vi "_Subscr.Ver Test Module2.vi"() -> ()   [LabVIEW 2024, in "EQMF.lvlib" / "Subscription.lvlib"]
uses:
  Subscription.lvlib
  Subscr.Subscription Request Info.ctl
  Queues/Q.Element.ctl
  Subscription.lvclass
  Queues/Queue Utils.lvlib
panel:
  out "SubScrReq":T1[](array[typedef])
  in  "stop":bool
  in  "Bool":bool
  in  "Str":string
  in  "Host Q":string="Module 1"
  out "Bool  Subsc":bool
  out "Str Subsc":string
  in  "Subscribe to Bool":bool
  in  "Subscribe to Str":bool
  in  "Local Q":string="Module 2"
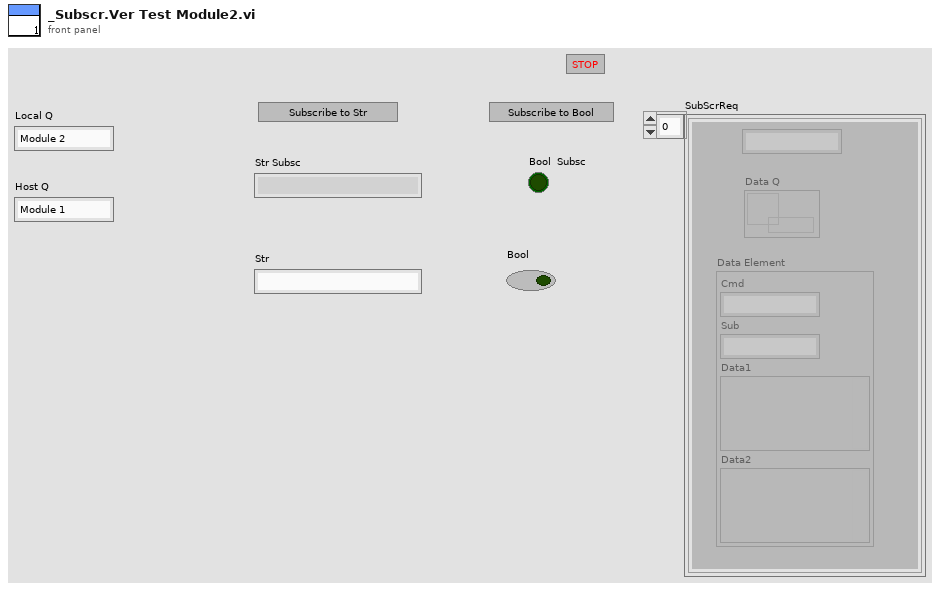
[diagram p1: front panel]
types:
  T1 = typedef "EQMF.lvlib/Subscription.lvlib/Subscr.Subscription Request Info.ctl" = cluster{"Name":string, "Data Q":refnum<queue>, "Data Element":T2}
  T2 = typedef "EQMF.lvlib/Queue Utils.lvlib/Q.Element.ctl" = cluster{"Cmd":string, "Sub":string, "Data1":variant, "Data2":variant}
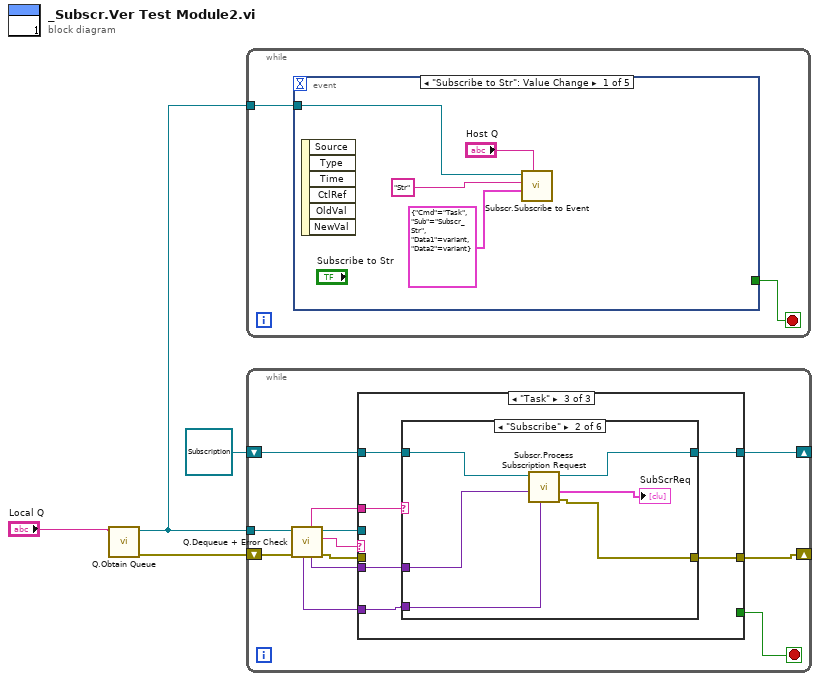
[diagram p0: block diagram]
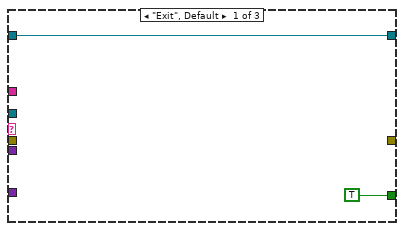
[diagram p2: hidden frame]
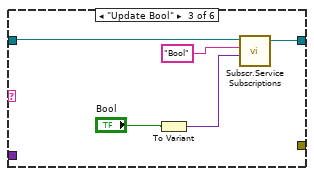
[diagram p5: hidden frame]
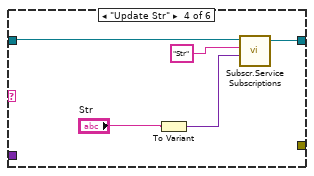
[diagram p6: hidden frame]
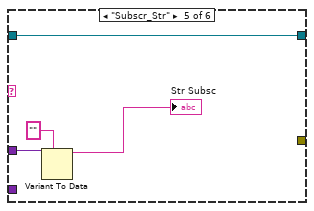
[diagram p7: hidden frame]
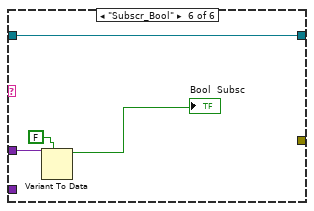
[diagram p8: hidden frame]
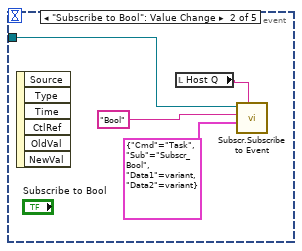
[diagram p9: hidden frame]
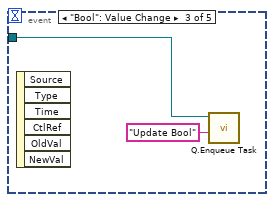
[diagram p10: hidden frame]
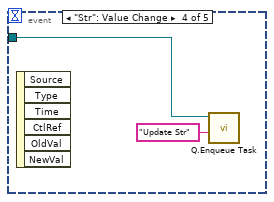
[diagram p11: hidden frame]
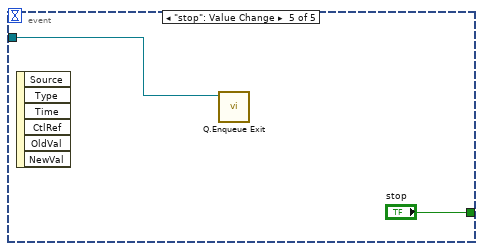
[diagram p12: hidden frame]
diagram:
  n1 = call "Q.Obtain Queue.vi"("Q Name"="Local Q") -> ("error out"=w1:errorcluster, "Q Out"=w3:refnum<queue>)  [unwired: 8 in, 1 out]
  n2 = while {
    tunnel: w3 -> [w6]
    stop <- w5 stop-if-true
    n3 = event shown="[0] \"Subscribe to Str\": Value Change" {
      selector: _ -> [_ _ _ _ _]
      dyn-events: _ -> [_ _ _ _ _]
      timeout: _ -> [_ _ _ _ _]
      tunnel: w6 -> [w10 w14 w16 w18 w19]
      tunnel: [_ _ _ _ "stop"] -> w5
      event "Subscribe to Str": Value Change {
        n4 = event-data() -> ()  [unwired: 1 in, 6 out]
        n5 = call "Subscr.Subscribe to Event.vi"("Source Q Name"="Host Q", "Data Element"=T2 {"Cmd"="Task", "Sub"="Subscr_Str", "Data1"=variant, "Data2"=variant}, "Event Name"="Str", "Local Q"=w10) -> ()  [unwired: 6 in, 2 out]
      }
      event "Subscribe to Bool": Value Change {
        n6 = event-data() -> ()  [unwired: 1 in, 6 out]
        n7 = local read "Host Q"() -> (w11:string)
        n8 = call "Subscr.Subscribe to Event.vi"("Source Q Name"=w11, "Data Element"=T2 {"Cmd"="Task", "Sub"="Subscr_Bool", "Data1"=variant, "Data2"=variant}, "Event Name"="Bool", "Local Q"=w14) -> ()  [unwired: 6 in, 2 out]
      }
      event "Bool": Value Change {
        n9 = event-data() -> ()  [unwired: 1 in, 6 out]
        n10 = call "Q.Enqueue Task.vi"("Task Name"="Update Bool", "Q In"=w16) -> ()  [unwired: 8 in, 2 out]
      }
      event "Str": Value Change {
        n11 = event-data() -> ()  [unwired: 1 in, 6 out]
        n12 = call "Q.Enqueue Task.vi"("Task Name"="Update Str", "Q In"=w18) -> ()  [unwired: 8 in, 2 out]
      }
      event "stop": Value Change {
        n13 = event-data() -> ()  [unwired: 1 in, 6 out]
        n14 = call "Q.Enqueue Exit.vi"("Q In"=w19) -> ()  [unwired: 9 in, 2 out]
      }
    }
  }
  n15 = while {
    tunnel: w3 -> [w32]
    shift-right: [w23] -> _
    shift-left: w1 -> [w24]
    shift-right: [w21] -> _
    shift-left: refnum<class "Subscription.lvclass"> refnum ("Subscription in") -> [w25]
    stop <- w26 stop-if-true
    n16 = call "Q.Dequeue + Error Check.vi"("Error In"=w24, "Q In"=w32) -> ("error out"=w22:errorcluster, "Cmd"=w30:string, "Q Out"=w31:refnum<queue>, "Data1"=w28:variant, "Sub"=w29:string, "Data2"=w27:variant)  [unwired: 4 in]
    n17 = case shown="\"Task\"" w30 {
      tunnel: w31 -> [_ _ _]
      tunnel: w29 -> [_ _ w41]
      tunnel: w28 -> [_ _ w40]
      tunnel: w27 -> [_ _ w36]
      tunnel: [TRUE _ _] -> w26
      tunnel: w25 -> [w33 w35 w39]
      tunnel: [_ _ w37] -> w23
      tunnel: w22 -> [_ _ _]
      tunnel: [w33 w35 w38] -> w21
      frame "Exit", Default {
      }
      frame "Error" {
      }
      frame "Task" {
        n18 = case shown="\"Subscribe\"" w41 {
          tunnel: w40 -> [_ w44 _ _ w62 w66]
          tunnel: w39 -> [w42 w48 w52 w57 w59 w63]
          tunnel: [w42 w47 w53 w58 w59 w63] -> w38
          tunnel: [_ w45 _ _ _ _] -> w37
          tunnel: w36 -> [_ w43 _ _ _ _]
          frame Default {
          }
          frame "Subscribe" {
            n19 = call "Subscr.Process Subscription Request.vi"("Disable(Data2)"=w43, "Request Info (Data1)"=w44, "Subscription in"=w48) -> ("error out"=w45:errorcluster, "SubScrReq"=→"SubScrReq":T1[], "Subscription out"=w47:refnum<class "Subscription.lvclass">)  [unwired: 6 in]
          }
          frame "Update Bool" {
            n20 = To Variant(anything="Bool") -> (Variant=w49:variant)
            n21 = call "Subscr.Service Subscriptions.vi"("Data"=w49, "Name"="Bool" ("Event Name"), "Subscription in"=w52) -> ("Subscription out"=w53:refnum<class "Subscription.lvclass">)  [unwired: 7 in, 1 out]
          }
          frame "Update Str" {
            n22 = To Variant(anything="Str") -> (Variant=w55:variant)
            n23 = call "Subscr.Service Subscriptions.vi"("Data"=w55, "Name"="Str" ("Event Name"), "Subscription in"=w57) -> ("Subscription out"=w58:refnum<class "Subscription.lvclass">)  [unwired: 7 in, 1 out]
          }
          frame "Subscr_Str" {
            n24 = Variant To Data(type="", Variant=w62) -> (data=→"Str Subsc":string)  [unwired: 1 in, 1 out]
          }
          frame "Subscr_Bool" {
            n25 = Variant To Data(type=FALSE ("Bool  Subsc"), Variant=w66) -> (data=→"Bool  Subsc":bool)  [unwired: 1 in, 1 out]
          }
        }
      }
    }
  }
